vi "表格单元格双色.vi"(8 "错误输入（无错误）":errorcluster, 9 "颜色":cluster{"原始颜色":u32, "选中颜色":u32}={"原始颜色"=16777216, "选中颜色"=16860}, 10 "坐标":T1={"Row"=20, "Column"=20} caption="本次坐标", 11 "引用输入":refnum<vi>) -> (0 "错误输出":errorcluster, 1 "改变颜色":bool, 2 "坐标输出":T1 caption="坐标", 3 "引用输出":refnum<vi>)   [LabVIEW 2014, in "表格.lvlib" / "表格上色.lvlib"]
uses:
  <vilib>/Utility/miscctls.llb/LVRowAndColumnTypeDef.ctl
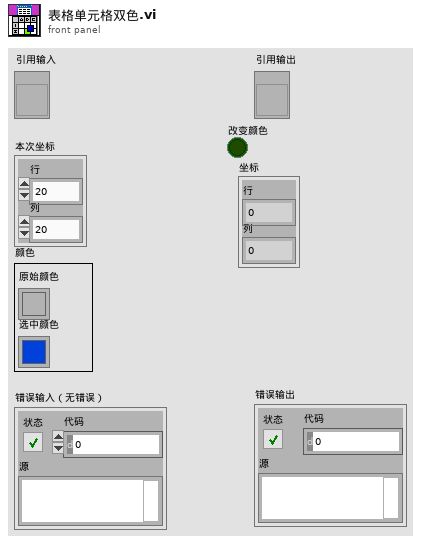
[diagram p1: front panel]
types:
  T1 = typedef "LVRowAndColumnTypeDef.ctl" = cluster{"Row":i32, "Column":i32}
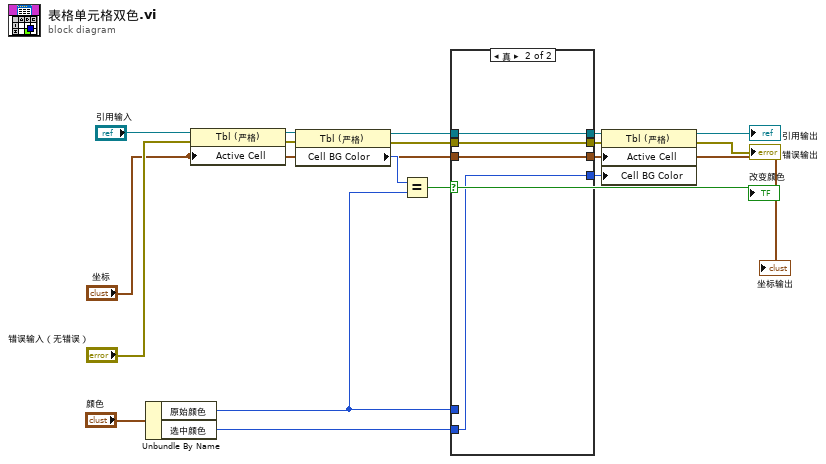
[diagram p0: block diagram]
diagram:
  n1 = Unbundle By Name("颜色") -> ("原始颜色"=w15:u32, "选中颜色"=w14:u32)
  n2 = property on="属性节点" class="Tbl (严格)"(reference="引用输入", error in="错误输入（无错误）", "Active Cell"="坐标") -> (reference out=w5:refnum<vi>, error out=w4:errorcluster)
  n3 = property on="属性节点" class="Tbl (严格)"(reference=w5, error in=w4) -> (reference out=w13:refnum<vi>, error out=w12:errorcluster, "Cell BG Color"=w11:u32)
  n4 = Equal?(x=w11, y=w15) -> (x = y?=w10:bool)
  "改变颜色" <- w10
  n5 = case shown="真" w10 {
    tunnel: [w21 w25] -> w8
    tunnel: "坐标" -> [w20 w24]
    tunnel: [w22 w26] -> w9
    tunnel: w13 -> [w22 w26]
    tunnel: w12 -> [w21 w25]
    tunnel: [w20 w24] -> w7
    tunnel: w14 -> [_ w23]
    tunnel: [w19 w23] -> w6
    tunnel: w15 -> [w19 _]
    frame False {
    }
    frame True {
    }
  }
  "坐标输出" <- w7
  n6 = property on="属性节点" class="Tbl (严格)"(reference=w9, error in=w8, "Active Cell"=w7, "Cell BG Color"=w6) -> (reference out=→"引用输出":refnum<vi>, error out=→"错误输出":errorcluster)
